vi "Main.vi"() -> ()   [LabVIEW 2017]
doc: "The myRIO Project template acquires acceleration data from the onboard accelerometer and displays the changes of acceleration values in a waveform chart."
uses:
  Working Demo Phase/states.ctl
  Working Demo Phase/Current Floor.ctl
  <vilib>/myRIO/Common/Instrument Driver Framework/myRIO v1.0/DIO/typedefs/DIO Channels Enum.ctl
  <vilib>/myRIO/Common/Instrument Driver Framework/myRIO v1.0/DIO/typedefs/DIO Channels List.ctl
  <vilib>/myRIO/Common/Instrument Driver Framework/Utilities/typedefs/Generic FPGA Reference.ctl
  <vilib>/myRIO/Common/Instrument Driver Framework/Utilities/typedefs/myRIO v1.0 Reference.ctl
  <vilib>/myRIO/Common/Instrument Driver Framework/Utilities/typedefs/Hardware Version Enum.ctl
  <vilib>/myRIO/Common/Instrument Driver Framework/Utilities/typedefs/myRIO Generic Hardware Reference.ctl
  <vilib>/myRIO/Instrument Drivers/Onboard IO/DIO/typedefs/DIO Reference.ctl
  <vilib>/myRIO/Instrument Drivers/Onboard IO/DIO/DIO.lvlib
  <vilib>/myRIO/Instrument Drivers/Onboard IO/DIO/vis/Read.vi
  <vilib>/userdefined/High Color/nirio_resource_hc.ctl
  <vilib>/myRIO/Common/Instrument Driver Framework/myRIO v1.0/DIO/vis/myRIO v1.1 Open DIO.vi
  <vilib>/myRIO/Instrument Drivers/Onboard IO/DIO/vis/myRIO DIO Open.xnode
  <vilib>/myRIO/Common/Instrument Driver Framework/Utilities/vis/Is FPGA Ref Available.vi
  <vilib>/myRIO/Express VI/Onboard IO/DI/DI Express VI.xnode
  <vilib>/myRIO/Instrument Drivers/Onboard IO/DIO/vis/Write.vi
  <vilib>/myRIO/Express VI/Onboard Devices/LED/LED Express VI.xnode
panel:
  out "Not Floor 1":bool
  out "Floor 1 OPTLIMSW (B/DIO1 (Pin 13))":bool
  out "Current State":T1
  out "Current Iteration":i32
  in  "Test Iterations":i32=1
  out "Written String 4":string
  out "Written String 3":string
  out "Written String 2":string
  out "Written String":string
  out "error out 2":errorcluster
  out "error out":errorcluster
  out "error out 5":errorcluster
  out "error out 4":errorcluster
  out "error out 3":errorcluster
  out "Floor Ground From Drop":i32
  out "Floor 1":i32
  out "Ground Floor":i32
  out "Floor 2":i32
  in  "Stop Button":bool
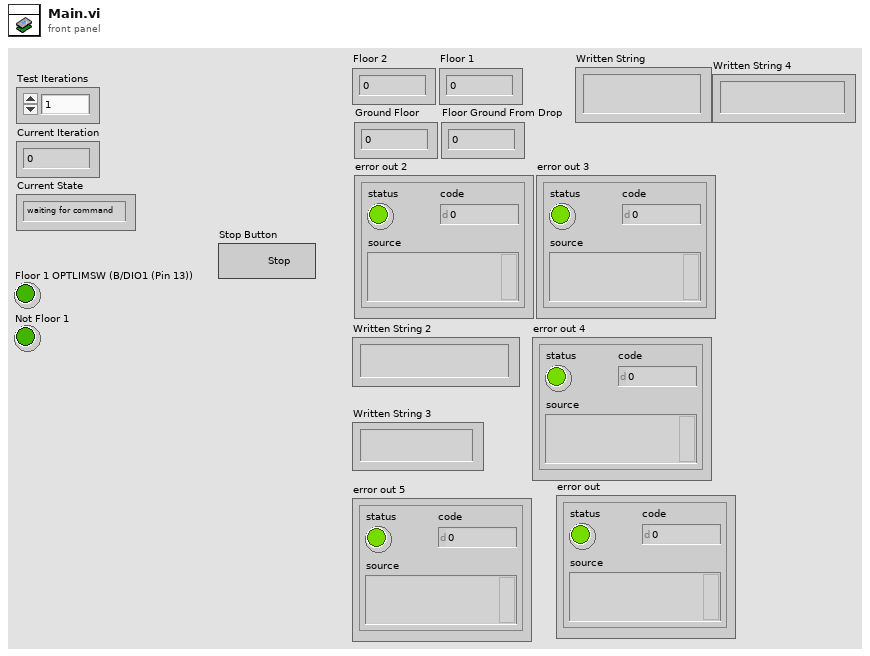
[diagram p1: front panel]
types:
  T1 = typedef "states.ctl" = enum16{"waiting for command", "go to ground floor", "go to floor 1", "go to floor 2", "drop cart"}
  T2 = enum16{"open", "replace", "create", "open or create", "replace or create", "replace or create with confirmation"}
  T3 = typedef "Current Floor.ctl" = enum16{"Ground Floor", "Floor 1", "Floor 2"}
  T4 = typedef "DIO.lvlib/DIO Reference.ctl" = cluster{"myRIO Reference":T5, "DIO Channels List":T9}
  T5 = typedef "myRIO Generic Hardware Reference.ctl" = cluster{"myRIO Model":T6, "myRIO Hardware Reference":T7}
  T6 = typedef "Hardware Version Enum.ctl" = enum16{"Unknown", "myRIO-1900", "myRIO-1950", "roboRIO", "NI ELVIS RIO CM"}
  T7 = typedef "myRIO v1.0 Reference.ctl" = cluster{"Generic FPGA Reference":T8, "Allow multiple opens":bool}
  T8 = typedef "Generic FPGA Reference.ctl" = refnum<k20>
  T9 = typedef "DIO Channels List.ctl" = T10[]
  T10 = typedef "DIO Channels Enum.ctl" = enum16{"Not Connected", "C/DIO0", "C/DIO1", "C/DIO2", "C/DIO3", "C/DIO4", "C/DIO5", "C/DIO6", "C/DIO7", "A/DIO0", "A/DIO1", "A/DIO2", "A/DIO3", "A/DIO4", "A/DIO5", "A/DIO6", "A/DIO7", "A/DIO8", "A/DIO9", "A/DIO10", "A/DIO11", "A/DIO12", "A/DIO13", "A/DIO14", "A/DIO15", "B/DIO0", "B/DIO1", "B/DIO2", "B/DIO3", "B/DIO4", "B/DIO5", "B/DIO6", "B/DIO7", "B/DIO8", "B/DIO9", "B/DIO10", "B/DIO11", "B/DIO12", "B/DIO13", "B/DIO14", "B/DIO15", "LED0", "LED1", "LED2", "LED3", "Button0", "DIO/DIO0", "DIO/DIO1", "DIO/DIO2", "DIO/DIO3", "DIO/DIO4", "DIO/DIO5", "DIO/DIO6", "DIO/DIO7", "DIO/DIO8", "DIO/DIO9", "SPI/CS0", "SPI/CS1", "SPI/CS2", "SPI/CS3", "LED RADIO (Green)", "LED RADIO (Red)", "LED COMM (Green)", "LED COMM (Red)", "LED MODE (Green)", "LED MODE (Red)"}
  T11 = typedef "nirio_resource_hc.ctl" = tag
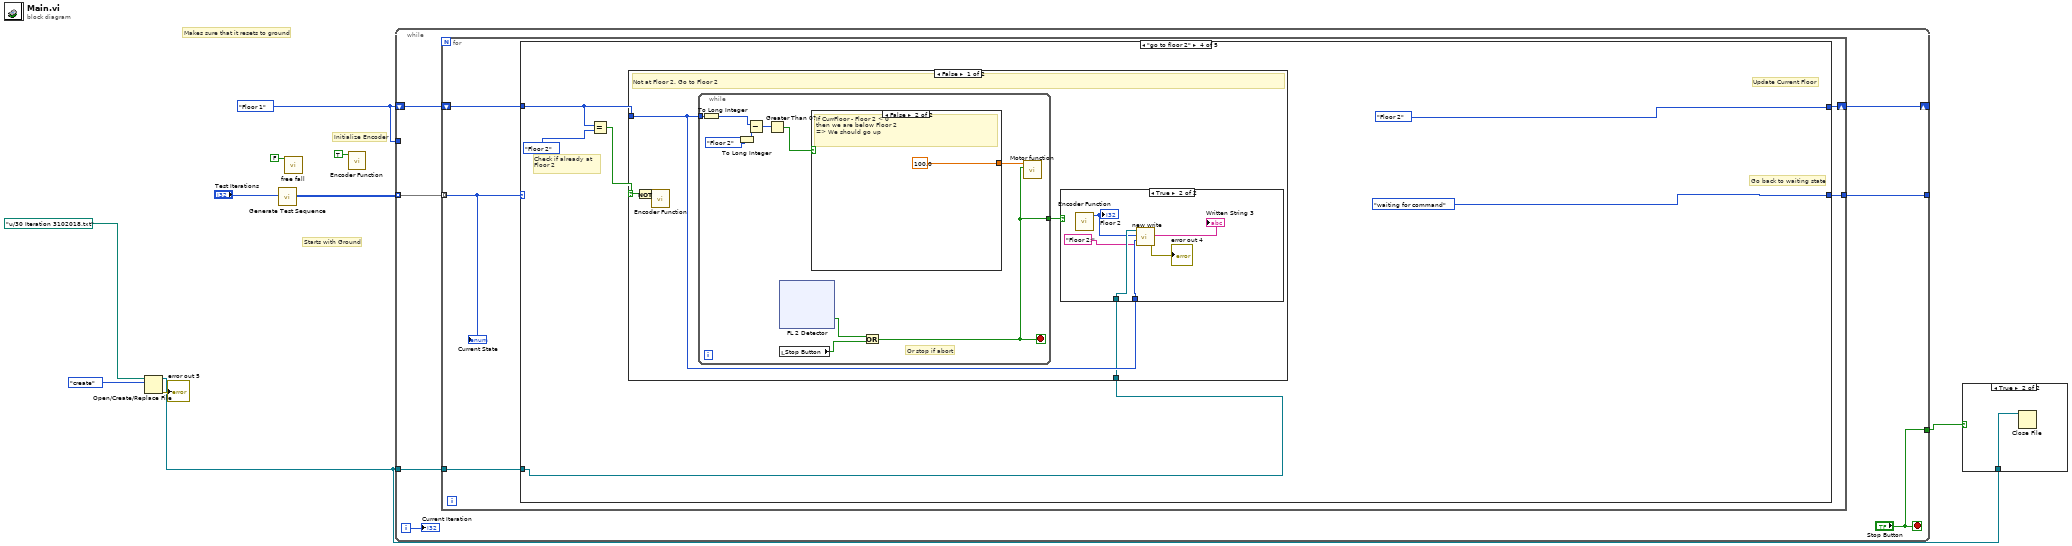
[diagram p0: block diagram]
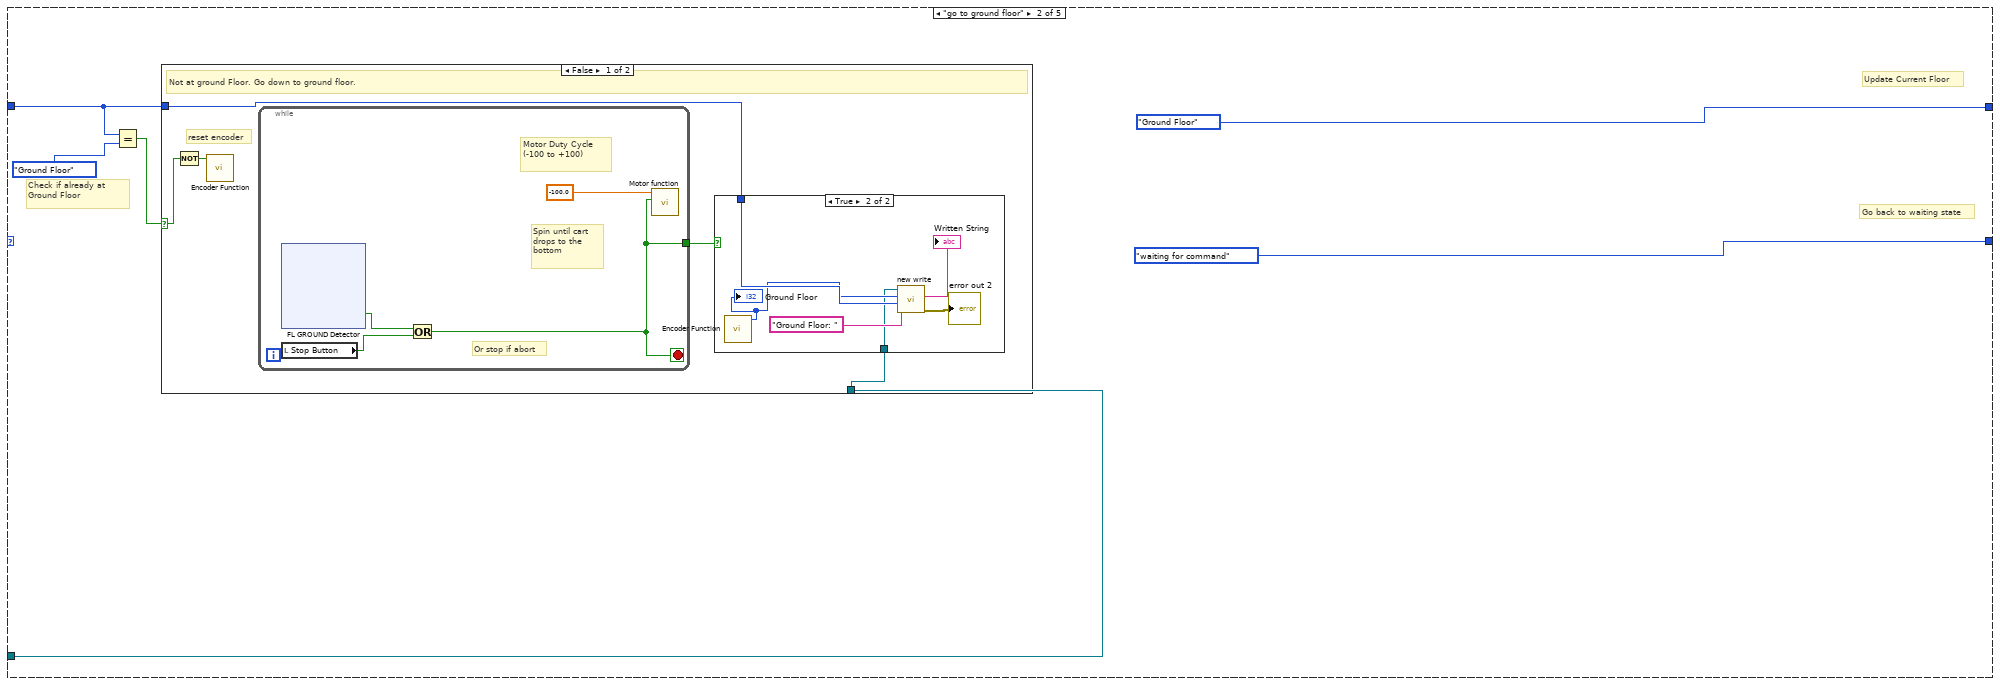
[diagram p4: hidden frame]
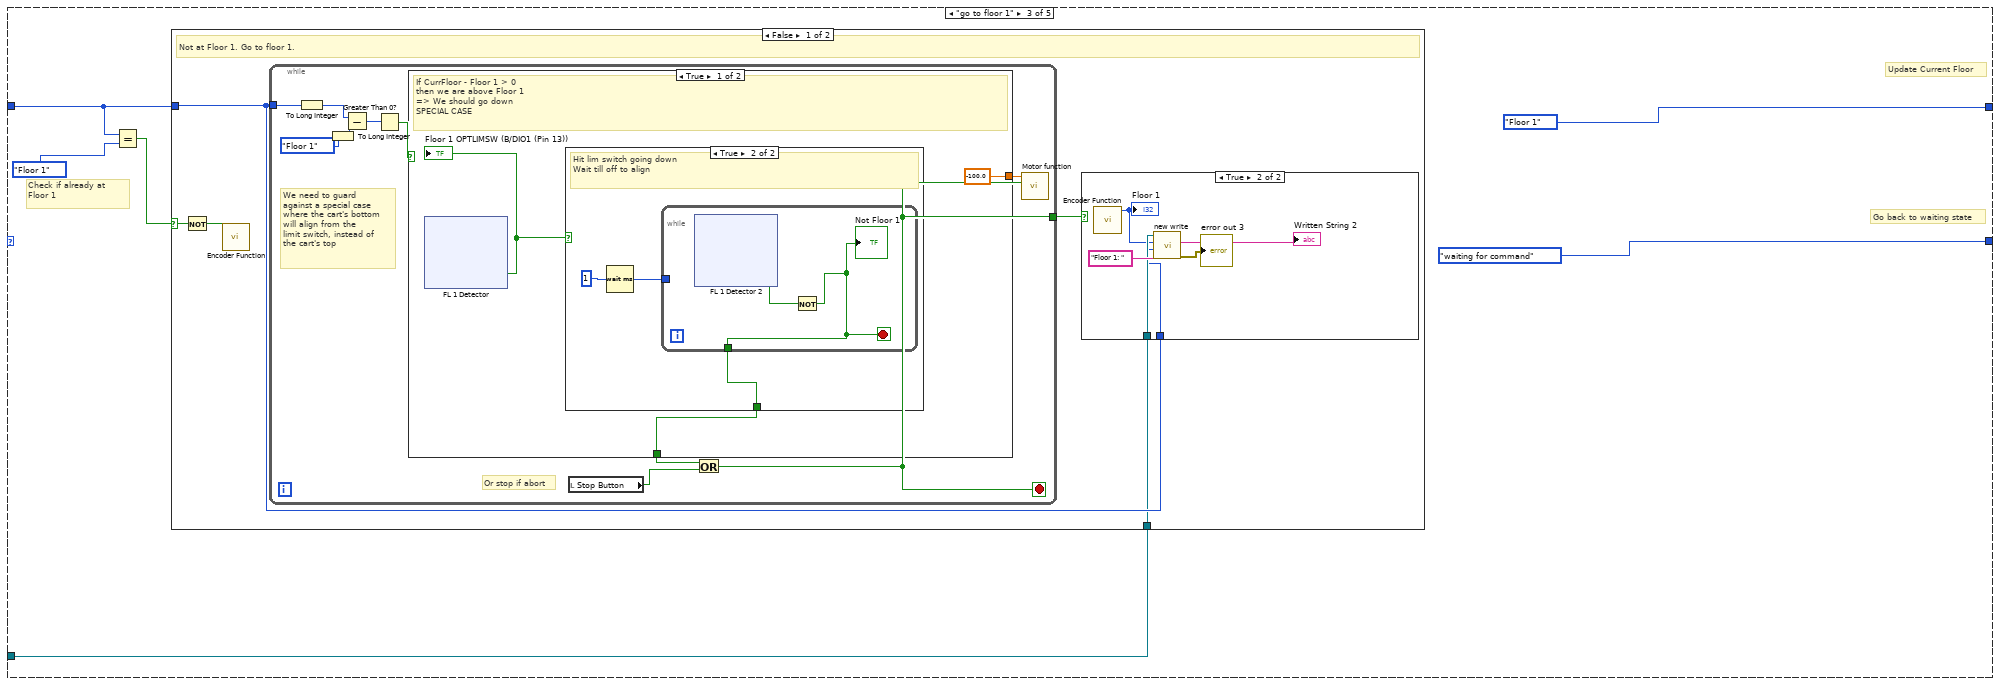
[diagram p7: hidden frame]
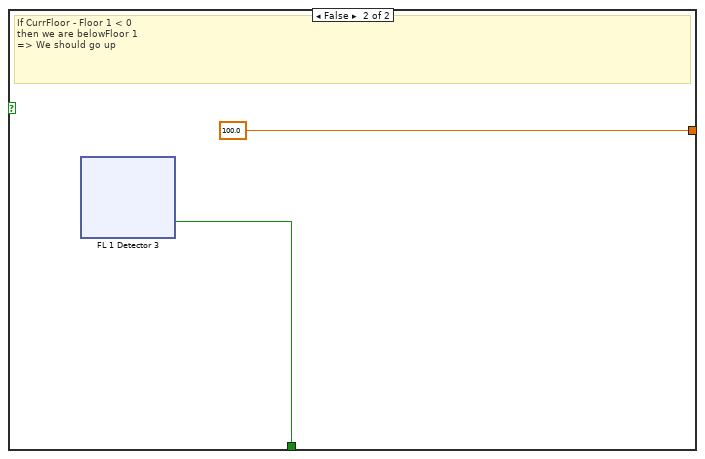
[diagram p10: hidden frame]
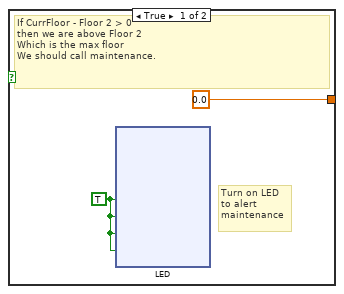
[diagram p13: hidden frame]
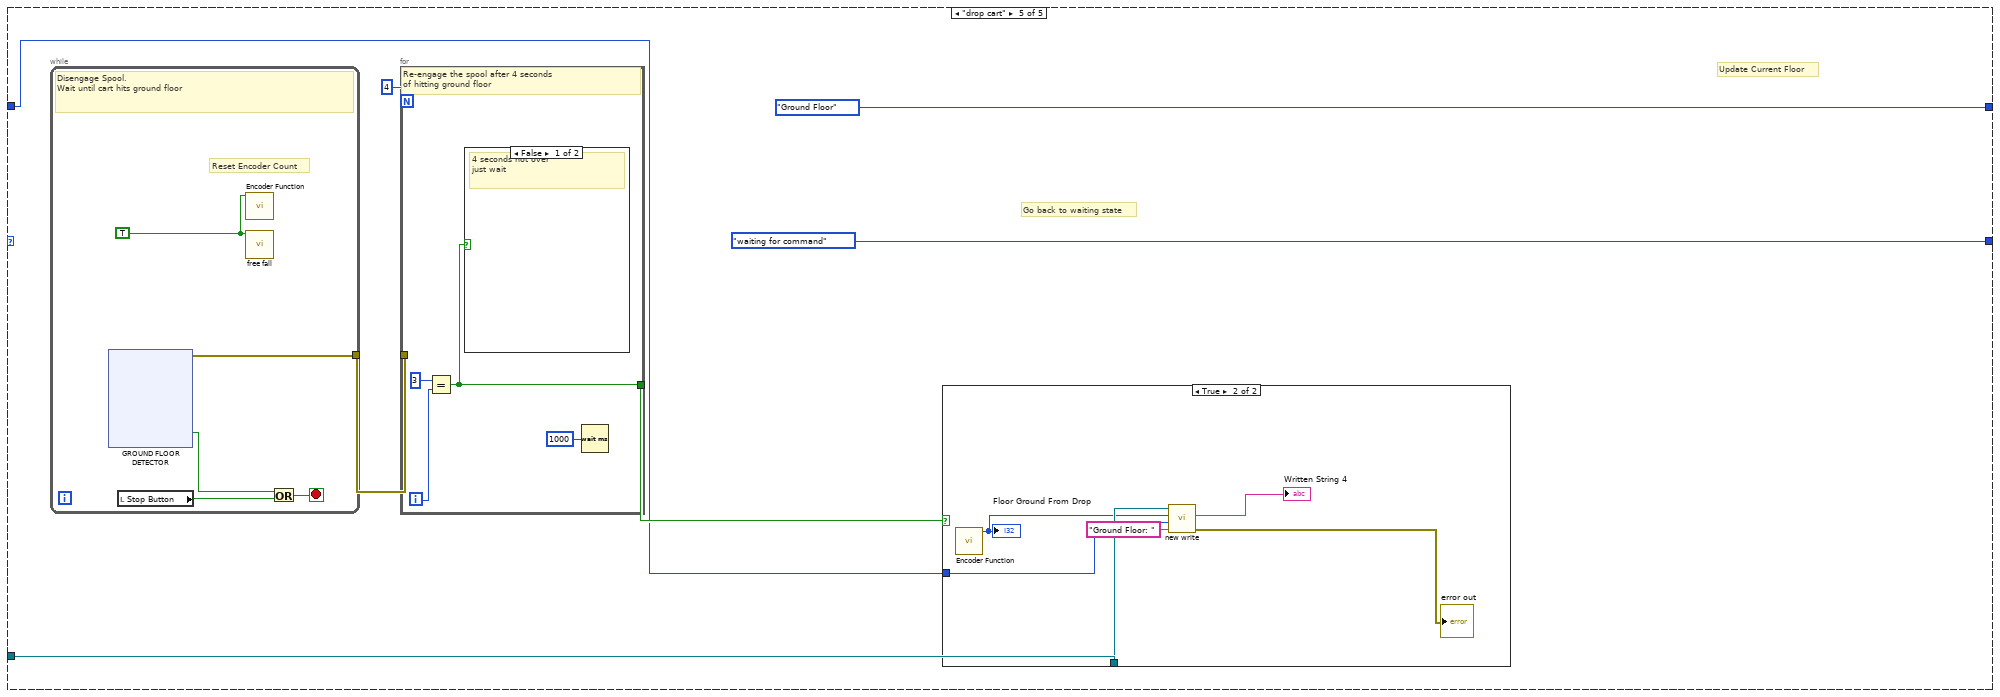
[diagram p15: hidden frame]
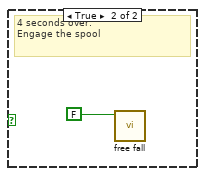
[diagram p17: hidden frame]
diagram:
  w7 = Current_Floor."Floor 1"
  # "Makes sure that it resets to ground"
  # "Starts with Ground"
  # "Initialize Encoder"
  n1 = Open/Create/Replace File(file path (use dialog)=path "u:/30 Iteration 3102018.txt", operation (0:open)=T2."create") -> (refnum out=w3:refnum<file>, error out=→"error out 5":errorcluster)  [unwired: 4 in, 1 out]
  n2 = call "Generate Test Sequence.vi"("Number of Iterations"="Test Iterations") -> ("Test Sequence"=w9:T1[][])  [unwired: 10 in]
  n3 = call "free fall.vi"("Freefall Button"=FALSE) -> ()  [unwired: 11 in]
  n4 = call "Encoder Function.vi"("Reset Counter in"=TRUE) -> ()  [unwired: 9 in, 2 out]
  n5 = while {
    shift-right: [w14] -> _
    shift-left: w7 -> [w15]
    tunnel: w9 -> [w17] mode=indexing
    tunnel: [w16] -> _
    tunnel: w7 -> [_]
    tunnel: w3 -> [w13]
    tunnel: ["Stop Button"] -> w2
    i -> [w11]
    stop <- "Stop Button" stop-if-true
    n6 = for {
      tunnel: w17 -> [w22] mode=indexing
      tunnel: [w21] -> w16
      shift-right: [w19] -> w14
      shift-left: w15 -> [w20]
      tunnel: w13 -> [w18]
      n7 = case shown="\"go to floor 2\"" w22 {
        selector: w22 -> [w23 _ _ _ _]
        tunnel: [w23 states."waiting for command" states."waiting for command" states."waiting for command" states."waiting for command"] -> w21
        tunnel: w20 -> [w24 w27 w83 w225 w327]
        tunnel: [w24 Current_Floor."Ground Floor" Current_Floor."Floor 1" Current_Floor."Floor 2" Current_Floor."Ground Floor"] -> w19
        tunnel: w18 -> [_ w25 w81 w223 w326]
        frame "waiting for command", Default {
        }
        frame "go to ground floor" {
          # "Update Current Floor"
          # "Go back to waiting state"
          # "Check if already at Ground Floor"
          n8 = Equal?(x=w27, y=Current_Floor."Ground Floor") -> (x = y?=w28:bool)
          n9 = case shown="False" w28 {
            selector: w28 -> [w35 _]
            tunnel: w27 -> [w32 _]
            tunnel: w25 -> [w31 _]
            frame False {
              # "reset encoder"
              # "Not at ground Floor. Go down to ground floor."
              n10 = Not(x=w35) -> (.not. x?=w33:bool)
              n11 = call "Encoder Function.vi"("Reset Counter in"=w33) -> ()  [unwired: 9 in, 2 out]
              n12 = while {
                tunnel: [w43] -> w34
                stop <- w43 stop-if-true
                # "Motor Duty Cycle (-100 to +100)"
                # "Or stop if abort"
                # "Spin until cart drops to the bottom"
                n13 = xnode "FL GROUND Detector"() -> ("Ground Floor OPTLIMSW (B/DIO3 (Pin 17))"=w44:bool)  [unwired: 1 in, 1 out]
                n14 = local read "Stop Button"() -> (w42:bool)
                n15 = Or(x=w44, y=w42) -> (x .or. y?=w43:bool)
                n16 = call "Motor function.vi"("Stop VI"=w43, "Duty Cycle (-100 to +100)"=-100.0) -> ()  [unwired: 10 in]
              }
              n17 = case shown="True" w34 {
                tunnel: w32 -> [_ w40]
                tunnel: w31 -> [_ w38]
                frame False {
                }
                frame True {
                  n18 = call "Encoder Function.vi"() -> ("Counter Value 2"=w39:i32)  [unwired: 10 in, 1 out]
                  "Ground Floor" <- w39
                  n19 = call "new write.vi"("Next Floor"="Ground Floor: ", "Current Floor"=w40, "Counter Value in"=w39, "Byte Stream File in"=w38) -> ("error out"=→"error out 2":errorcluster, "Written String"=→"Written String":string)  [unwired: 6 in]
                }
              }
            }
            frame True {
              # "Already at Ground Floor. Do nothing"
            }
          }
        }
        frame "go to floor 1" {
          # "Update Current Floor"
          # "Go back to waiting state"
          # "Check if already at Floor 1"
          n20 = Equal?(x=w83, y=Current_Floor."Floor 1") -> (x = y?=w84:bool)
          n21 = case shown="False" w84 {
            selector: w84 -> [w91 _]
            tunnel: w83 -> [w88 _]
            tunnel: w81 -> [w87 _]
            frame False {
              # "Not at Floor 1. Go to floor 1."
              n22 = Not(x=w91) -> (.not. x?=w90:bool)
              n23 = call "Encoder Function.vi"("Reset Counter in"=w90) -> ()  [unwired: 9 in, 2 out]
              n24 = while {
                tunnel: w88 -> [w107]
                tunnel: [w100] -> w89
                stop <- w100 stop-if-true
                # "We need to guard\nagainst a special case\nwhere the cart's bottom\nwill align from the\nlimit switch, instead of\nthe cart's top"
                # "Or stop if abort"
                n25 = To Long Integer(number=w107) -> (32bit integer=w102:i32)
                n26 = To Long Integer(number=Current_Floor."Floor 1") -> (32bit integer=w101:i32)
                n27 = Subtract(x=w102, y=w101) -> (x-y=w105:i32)
                n28 = Greater Than 0?(x=w105) -> (x > 0?=w104:bool)
                n29 = case shown="True" w104 {
                  tunnel: [-100.0 ("Duty Cycle (-100 to +100)") 100.0 ("Duty Cycle (-100 to +100)")] -> w103
                  tunnel: [w108 w186] -> w98
                  frame True {
                    # "If CurrFloor - Floor 1 > 0\nthen we are above Floor 1\n=> We should go down\nSPECIAL CASE"
                    n30 = xnode "FL 1 Detector"() -> ("Floor 1 OPTLIMSW (B/DIO1 (Pin 13))"=w109:bool)  [unwired: 1 in, 1 out]
                    "Floor 1 OPTLIMSW (B/DIO1 (Pin 13))" <- w109
                    n31 = case shown="True" w109 {
                      tunnel: [_ w113] -> w108
                      frame False {
                      }
                      frame True {
                        # "Hit lim switch going down\nWait till off to align"
                        n32 = Wait (ms)(milliseconds to wait=u32 1) -> (millisecond timer value=w111:u32)
                        n33 = while {
                          tunnel: [w114] -> w113
                          tunnel: w111 -> [_]
                          stop <- w114 stop-if-true
                          n34 = xnode "FL 1 Detector 2"() -> ("Floor 1 OPTLIMSW (B/DIO1 (Pin 13))"=w115:bool)  [unwired: 1 in, 1 out]
                          n35 = Not(x=w115) -> (.not. x?=w114:bool)
                          "Not Floor 1" <- w114
                        }
                      }
                    }
                  }
                  frame False {
                    # "If CurrFloor - Floor 1 < 0\nthen we are belowFloor 1\n=> We should go up"
                    n36 = xnode "FL 1 Detector 3"() -> ("Floor 1 OPTLIMSW (B/DIO1 (Pin 13))"=w186:bool)  [unwired: 1 in, 1 out]
                  }
                }
                n37 = local read "Stop Button"() -> (w99:bool)
                n38 = Or(x=w98, y=w99) -> (x .or. y?=w100:bool)
                n39 = call "Motor function.vi"("Stop VI"=w100, "Duty Cycle (-100 to +100)"=w103) -> ()  [unwired: 10 in]
              }
              n40 = case shown="True" w89 {
                tunnel: w88 -> [_ w93]
                tunnel: w87 -> [_ w95]
                frame False {
                }
                frame True {
                  n41 = call "Encoder Function.vi"() -> ("Counter Value 2"=w94:i32)  [unwired: 10 in, 1 out]
                  "Floor 1" <- w94
                  n42 = call "new write.vi"("Next Floor"="Floor 1: ", "Current Floor"=w93, "Counter Value in"=w94, "Byte Stream File in"=w95) -> ("error out"=→"error out 3":errorcluster, "Written String"=→"Written String 2":string)  [unwired: 6 in]
                }
              }
            }
            frame True {
              # "Already at Floor 1. Do nothing"
            }
          }
        }
        frame "go to floor 2" {
          # "Update Current Floor"
          # "Go back to waiting state"
          # "Check if already at Floor 2"
          n43 = Equal?(x=w225, y=Current_Floor."Floor 2") -> (x = y?=w226:bool)
          n44 = case shown="False" w226 {
            selector: w226 -> [w232 _]
            tunnel: w225 -> [w230 _]
            tunnel: w223 -> [w229 _]
            frame False {
              # "Not at Floor 2. Go to Floor 2"
              n45 = Not(x=w232) -> (.not. x?=w231:bool)
              n46 = call "Encoder Function.vi"("Reset Counter in"=w231) -> ()  [unwired: 9 in, 2 out]
              n47 = while {
                tunnel: w230 -> [w249]
                tunnel: [w241] -> w233
                stop <- w241 stop-if-true
                # "Or stop if abort"
                n48 = To Long Integer(number=w249) -> (32bit integer=w244:i32)
                n49 = To Long Integer(number=Current_Floor."Floor 2") -> (32bit integer=w243:i32)
                n50 = Subtract(x=w244, y=w243) -> (x-y=w247:i32)
                n51 = Greater Than 0?(x=w247) -> (x > 0?=w246:bool)
                n52 = xnode "FL 2 Detector"() -> ("Floor 2 OPTLIMSW (B/DIO2 (Pin 15))"=w242:bool)  [unwired: 1 in, 1 out]
                n53 = local read "Stop Button"() -> (w240:bool)
                n54 = case shown="False" w246 {
                  tunnel: [0.0 ("Duty Cycle (-100 to +100)") 100.0 ("Duty Cycle (-100 to +100)")] -> w245
                  frame True {
                    w250 = TRUE ("LED0")
                    # "Turn on LED\nto alert\nmaintenance"
                    # "If CurrFloor - Floor 2 > 0\nthen we are above Floor 2\nWhich is the max floor\nWe should call maintenance."
                    n55 = xnode "LED"("LED0"=w250, "LED1"=w250, "LED2"=w250, "LED3"=w250) -> ()  [unwired: 1 in, 1 out]
                  }
                  frame False {
                    # "If CurrFloor - Floor 2 < 0\nthen we are below Floor 2\n=> We should go up"
                  }
                }
                n56 = Or(x=w242, y=w240) -> (x .or. y?=w241:bool)
                n57 = call "Motor function.vi"("Stop VI"=w241, "Duty Cycle (-100 to +100)"=w245) -> ()  [unwired: 10 in]
              }
              n58 = case shown="True" w233 {
                tunnel: w230 -> [_ w237]
                tunnel: w229 -> [_ w238]
                frame False {
                }
                frame True {
                  n59 = call "Encoder Function.vi"() -> ("Counter Value 2"=w236:i32)  [unwired: 10 in, 1 out]
                  "Floor 2" <- w236
                  n60 = call "new write.vi"("Next Floor"="Floor 2:", "Current Floor"=w237, "Counter Value in"=w236, "Byte Stream File in"=w238) -> ("error out"=→"error out 4":errorcluster, "Written String"=→"Written String 3":string)  [unwired: 6 in]
                }
              }
            }
            frame True {
              # "Already at Floor 2. Do nothing"
            }
          }
        }
        frame "drop cart" {
          # "Update Current Floor"
          # "Go back to waiting state"
          n61 = while {
            tunnel: [w347] -> w331
            stop <- w348 stop-if-true
            w345 = TRUE
            # "Reset Encoder Count"
            # "Disengage Spool.\nWait until cart hits ground floor"
            n62 = xnode "GROUND FLOOR DETECTOR"() -> ("GROUND FL OPTLIMSW (B/DIO3 (Pin 17))"=w346:bool, "error out"=w347:errorcluster)  [unwired: 1 in]
            n63 = local read "Stop Button"() -> (w344:bool)
            n64 = call "Encoder Function.vi"("Reset Counter in"=w345) -> ()  [unwired: 9 in, 2 out]
            n65 = call "free fall.vi"("Freefall Button"=w345) -> ()  [unwired: 11 in]
            n66 = Or(x=w346, y=w344) -> (x .or. y?=w348:bool)
          }
          n67 = for {
            N: 4 -> [_]
            tunnel: w331 -> [_]
            tunnel: [w339] -> w328
            i -> [w342]
            # "Re-engage the spool after 4 seconds \nof hitting ground floor"
            n68 = Equal?(x=3, y=w342) -> (x = y?=w339:bool)
            n69 = case shown="False" w339 {
              frame False {
                # "4 seconds not over\njust wait"
              }
              frame True {
                # "4 seconds over.\nEngage the spool"
                n70 = call "free fall.vi"("Freefall Button"=FALSE) -> ()  [unwired: 11 in]
              }
            }
            n71 = Wait (ms)(milliseconds to wait=u32 1000) -> ()  [unwired: 1 out]
          }
          n72 = case shown="True" w328 {
            tunnel: w327 -> [_ w338]
            tunnel: w326 -> [_ w337]
            frame False {
            }
            frame True {
              n73 = call "Encoder Function.vi"() -> ("Counter Value 2"=w336:i32)  [unwired: 10 in, 1 out]
              "Floor Ground From Drop" <- w336
              n74 = call "new write.vi"("Next Floor"="Ground Floor: ", "Current Floor"=w338, "Counter Value in"=w336, "Byte Stream File in"=w337) -> ("error out"=→"error out":errorcluster, "Written String"=→"Written String 4":string)  [unwired: 6 in]
            }
          }
        }
      }
      "Current State" <- w22
    }
    "Current Iteration" <- w11
  }
  n75 = case shown="True" w2 {
    tunnel: w3 -> [_ w384]
    frame False {
    }
    frame True {
      n76 = Close File(refnum=w384) -> ()  [unwired: 1 in, 2 out]
    }
  }
